vi "GET Model.vi"(8 "error in":errorcluster) -> (0 "error out":errorcluster, 2 "Model Names":string[](array[string]))   [LabVIEW 2013]
uses:
  <vilib>/addons/database/Connection.llb/DB Tools Open Connec (String).vi
  <vilib>/addons/database/Connection.llb/Conn Execute.vi
  <vilib>/addons/database/Recordset.llb/Rec Fetch Recordset Data (R).vi
  <vilib>/addons/database/Recordset.llb/Rec Destroy - Connection.vi
  <vilib>/addons/database/NI_Database_API.lvlib
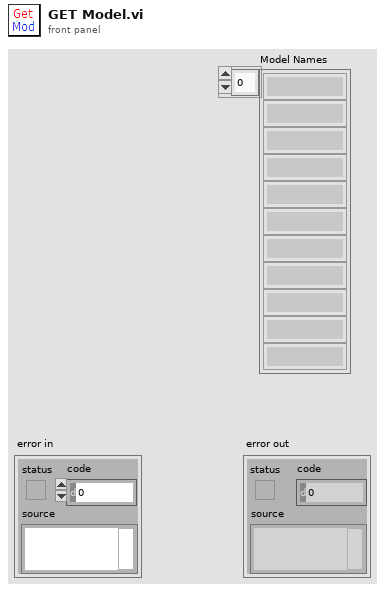
[diagram p1: front panel]
types:
  T1 = typedef "NI_Database_API.lvlib/Conn ObjectReference.ctl" = refnum<k1>
  T2 = typedef "NI_Database_API.lvlib/Rec ObjectReference.ctl" = refnum<k1>
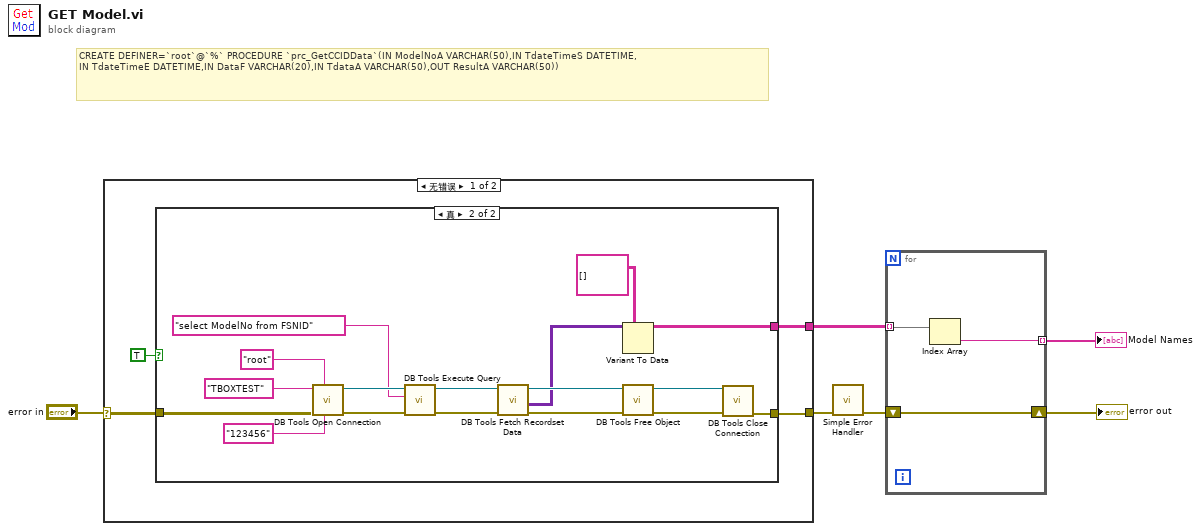
[diagram p0: block diagram]
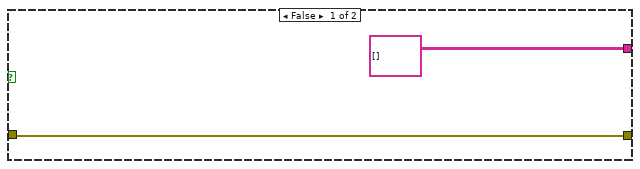
[diagram p2: hidden frame]
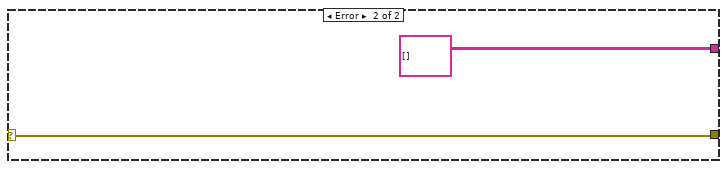
[diagram p3: hidden frame]
diagram:
  # "CREATE DEFINER=`root`@`%` PROCEDURE `prc_GetCCIDData`(IN ModelNoA VARCHAR(50),IN TdateTimeS DATETIME,\nIN TdateTimeE DATETIME,IN DataF VARCHAR(20),IN TdataA VARCHAR(50),OUT ResultA VARCHAR(50))"
  n1 = case shown="无错误" "error in" {
    selector: "error in" -> [w8 w31]
    tunnel: [w10 w31] -> w6
    tunnel: [w9 string[][] []] -> w4
    frame No Error {
      n2 = case shown="真" TRUE {
        tunnel: [w12 w23] -> w10
        tunnel: [string[][] [] w16] -> w9
        tunnel: w8 -> [w12 w15]
        frame False {
        }
        frame True {
          n3 = call-poly <vilib>:"DB Tools Open Connection.vi"("password"="123456", "userID"="root", "error in (no error)"=w15, "connection information"="TBOXTEST") -> ("error out"=w27:errorcluster, "connection reference"=w26:T1)  [unwired: 4 in]
          n4 = call-poly <vilib>:"DB Tools Execute Query.vi"("error in (no error)"=w27, "SQL query"="select ModelNo from FSNID", "connection reference"=w26) -> ("error out"=w24:errorcluster, "recordset reference"=w25:T2)  [unwired: 5 in]
          n5 = call-poly <vilib>:"DB Tools Fetch Recordset Data.vi"("error in (no error)"=w24, "recordset reference"=w25) -> ("error out"=w22:errorcluster, "recordset data"=w18:variant[][], "recordset reference out"=w21:T2)  [unwired: 3 in]
          n6 = Variant To Data(type=string[][] [], Variant=w18) -> (data=w16:string[][])  [unwired: 1 in, 1 out]
          n7 = call-poly <vilib>:"DB Tools Free Object.vi"("error in (no error)"=w22, "recordset reference"=w21) -> ("error out"=w20:errorcluster, "connection reference"=w19:T1)  [unwired: 8 in]
          n8 = call <vilib>:"DB Tools Close Connection.vi"("error in (no error)"=w20, "connection reference"=w19) -> ("error out"=w23:errorcluster)  [unwired: 5 in]
        }
      }
    }
    frame Error {
    }
  }
  n9 = call <vilib>:"Simple Error Handler.vi"("error in (no error)"=w6) -> ("error out"=w2:errorcluster)  [unwired: 4 in, 4 out]
  n10 = for {
    tunnel: w4 -> [w33] mode=indexing
    shift-right: [w34] -> w3
    shift-left: w2 -> [w34]
    tunnel: [w32] -> w1 mode=indexing
    n11 = Index Array(array=w33) -> (element=w32:string)  [unwired: 1 in]
  }
  "error out" <- w3
  "Model Names" <- w1
